vi "Zoe.prod.cons.vi"() -> ()   [LabVIEW 2014]
uses:
  Stack_State.ctl
  Stack Track.ctl
  Zoe_State.ctl
  PiFOC/PiFOC State.ctl
  <vilib>/vision/NI_Vision_Development_Module.lvlib
panel:
  in  "Move Piezo":bool
  out "Z Estimation":sgl(graph)
  in  "Template Path  2":path
  in  "Template Path":path
  out "Y Guess":dbl
  out "X Guess":dbl
  in  "Centroid Update":bool
  out "Cropped Image":T1(plugin-control)
  out "Raw Image":T1(plugin-control)
  in  "ROI Radius":dbl
  in  "Y Guess":dbl
  in  "X Guess":dbl
  out "Y Centroid":sgl
  out "X Centroid":sgl
  out "error out":errorcluster
  in  "stop":bool
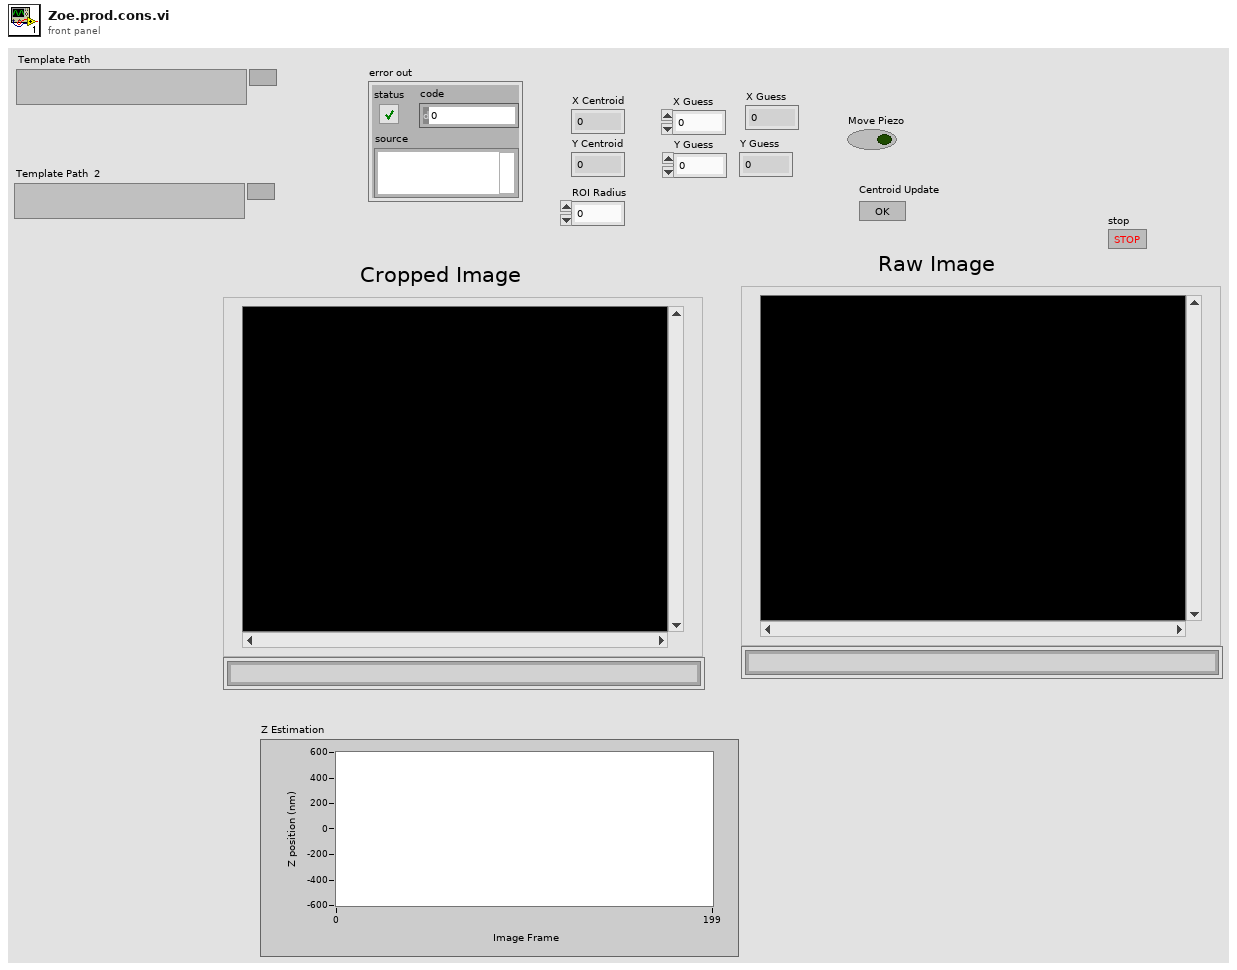
[diagram p1: front panel]
types:
  T1 = typedef "IMAQ Image.ctl" = refnum<image>
  T2 = typedef "PiFOC State.ctl" = enum16{"Idle", "GoTo", "getPosition"}
  T3 = typedef "Image Type" = u32
  T4 = typedef "Zoe_State.ctl" = enum16{"Centroid Update", "Idle", "Preview"}
  T5 = typedef "Stack_State.ctl" = cluster{"State":T6, "Stack Number":i32, "Image":u16[][], "Stacks":i32}
  T6 = typedef "Stack Track.ctl" = enum16{"Idle", "Preview", "Start Sequence", "Read Disk", "STOP", "Collecting", "End"}
  T7 = cluster{"Mean Value":sgl, "Standard Variation":sgl, "Minimal Value":sgl, "Maximal Value":sgl, "Area (calibrated)":sgl, "Area (pixels)":u32, "%":sgl, "Calibration Valid":bool}
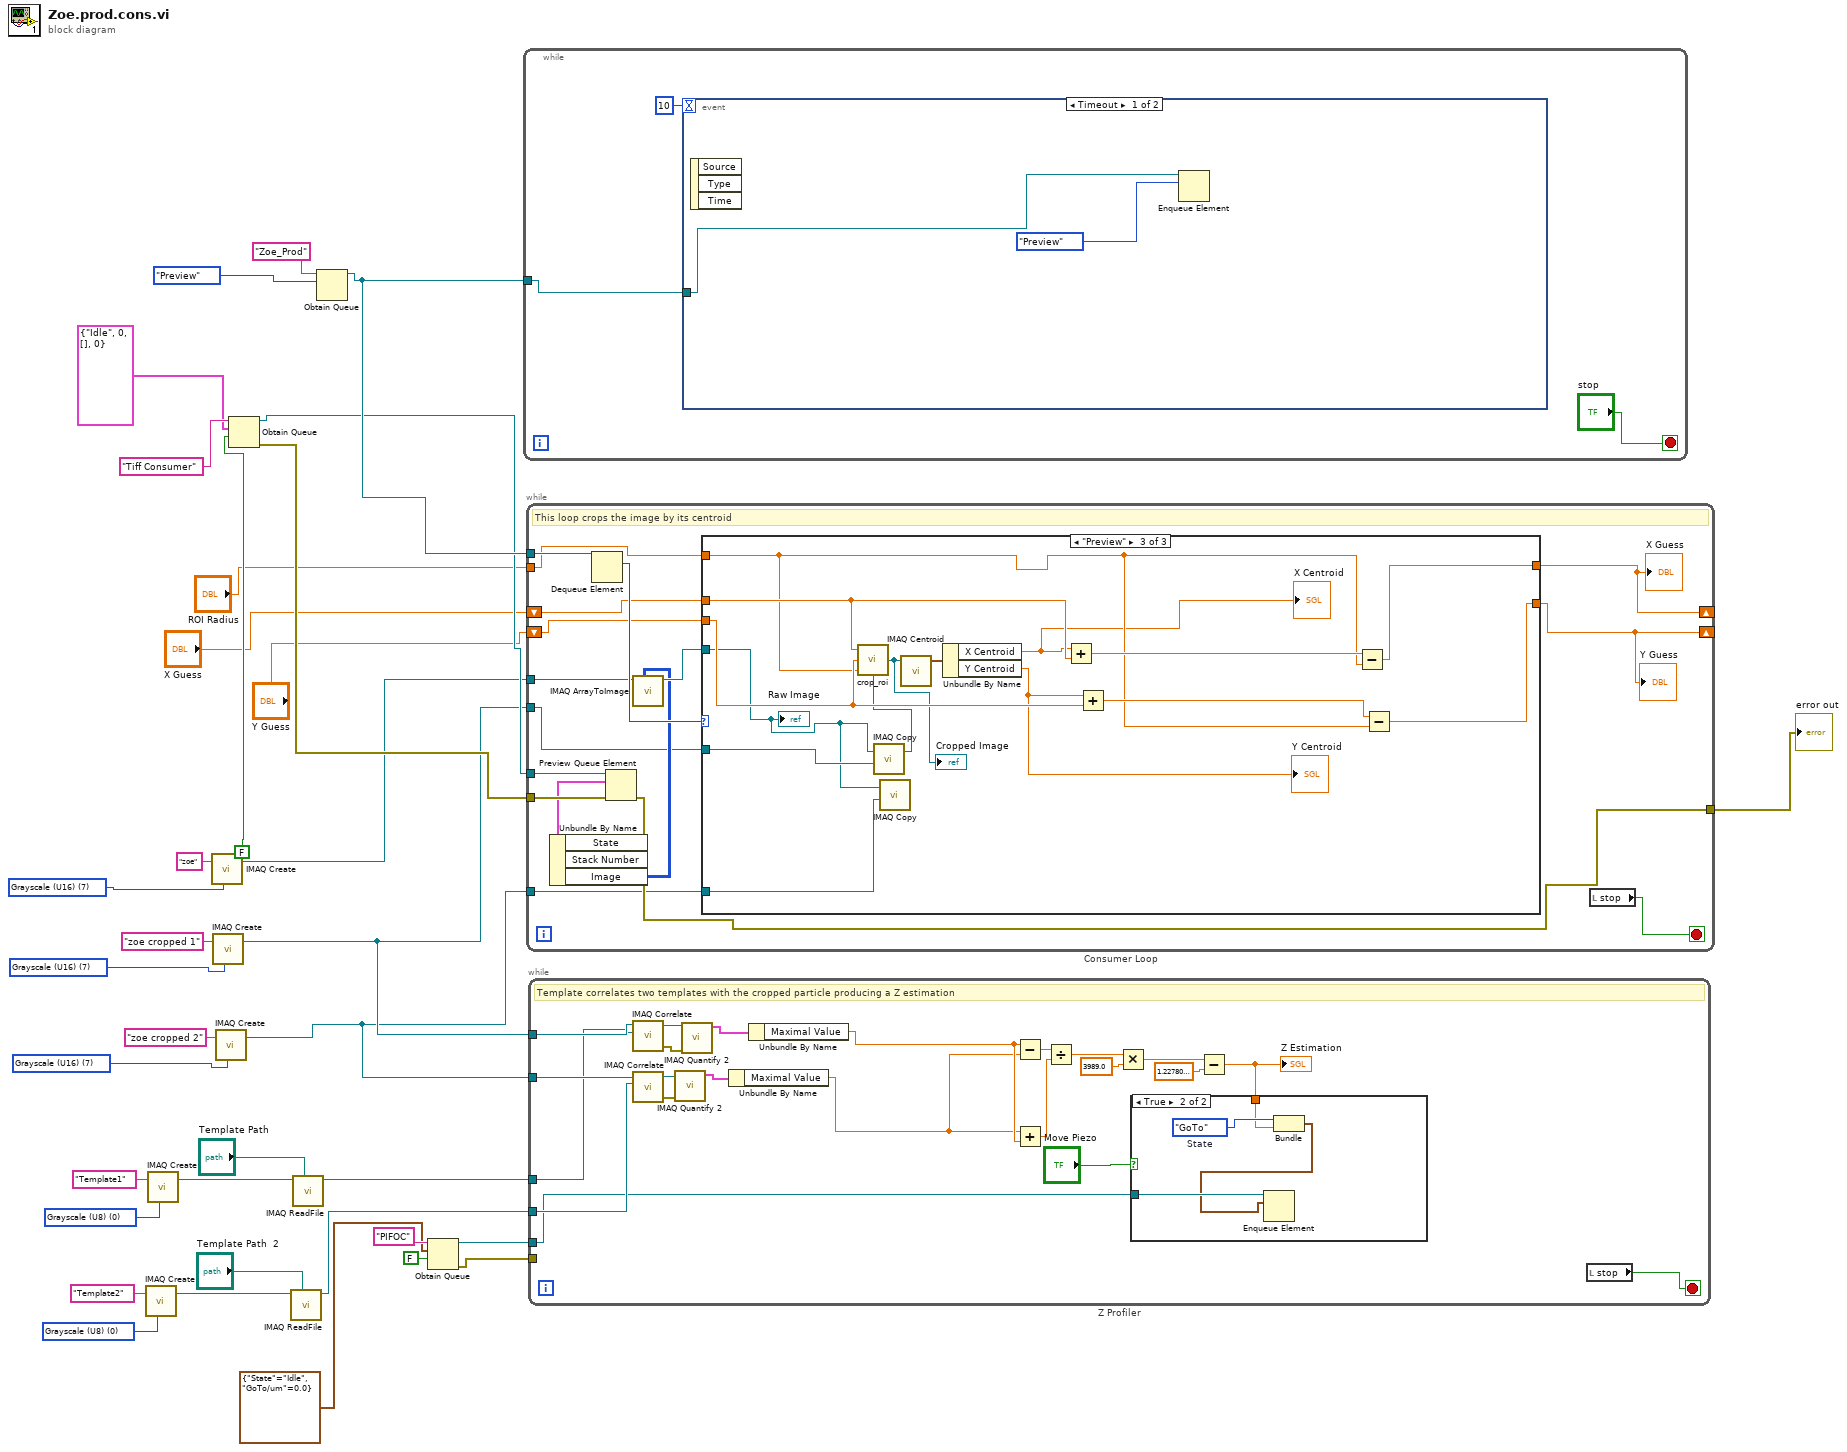
[diagram p0: block diagram]
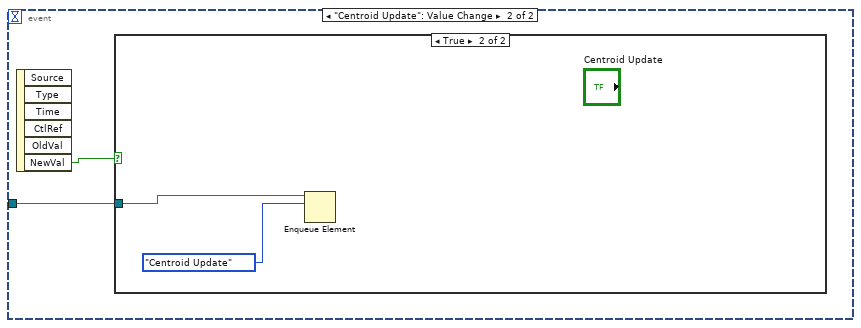
[diagram p5: hidden frame]
diagram:
  w8 = T3 0 items=["Grayscale (U8)", "Grayscale (I16)", "Grayscale (SGL)", "Complex (CSG)", "RGB (U32)", "HSL (U32)", "RGB (U64)", "Grayscale (U16)"] ("Image Type")
  w15 = T3 0 items=["Grayscale (U8)", "Grayscale (I16)", "Grayscale (SGL)", "Complex (CSG)", "RGB (U32)", "HSL (U32)", "RGB (U64)", "Grayscale (U16)"] ("Image Type")
  w18 = T3 7 items=["Grayscale (U8)", "Grayscale (I16)", "Grayscale (SGL)", "Complex (CSG)", "RGB (U32)", "HSL (U32)", "RGB (U64)", "Grayscale (U16)"] ("Image Type")
  w20 = T3 7 items=["Grayscale (U8)", "Grayscale (I16)", "Grayscale (SGL)", "Complex (CSG)", "RGB (U32)", "HSL (U32)", "RGB (U64)", "Grayscale (U16)"] ("Image Type")
  w23 = T3 7 items=["Grayscale (U8)", "Grayscale (I16)", "Grayscale (SGL)", "Complex (CSG)", "RGB (U32)", "HSL (U32)", "RGB (U64)", "Grayscale (U16)"] ("Image Type")
  n1 = call "IMAQ Create"("Image Name"="Template2", "Image Type"=w8) -> ("New Image"=w10:T1)  [unwired: 3 in, 1 out]
  n2 = call "IMAQ Create"("Image Name"="Template1", "Image Type"=w15) -> ("New Image"=w13:T1)  [unwired: 3 in, 1 out]
  n3 = call "IMAQ Create"("Image Name"="zoe", "Image Type"=w23) -> ("New Image"=w24:T1)  [unwired: 3 in, 1 out]
  n4 = call "IMAQ Create"("Image Name"="zoe cropped 1", "Image Type"=w20) -> ("New Image"=w19:T1)  [unwired: 3 in, 1 out]
  n5 = call "IMAQ Create"("Image Name"="zoe cropped 2", "Image Type"=w18) -> ("New Image"=w16:T1)  [unwired: 3 in, 1 out]
  n6 = Obtain Queue(name (unnamed)="Tiff Consumer", element data type=T5 {"State"=enum."Idle", "Stack Number"=0, "Image"=[], "Stacks"=0} ("input cluster"), create if not found? (T)=FALSE) -> (queue out=w30:refnum<queue>, error out=w29:errorcluster)  [unwired: 2 in, 1 out]
  n7 = call "IMAQ ReadFile"("File Path"="Template Path  2", "Image"=w10) -> ("Image Out"=w6:T1)  [unwired: 5 in, 4 out]
  n8 = call "IMAQ ReadFile"("File Path"="Template Path", "Image"=w13) -> ("Image Out"=w7:T1)  [unwired: 5 in, 4 out]
  n9 = Obtain Queue(name (unnamed)="Zoe_Prod", element data type=Zoe_State."Preview") -> (queue out=w31:refnum<queue>)  [unwired: 3 in, 2 out]
  n10 = Obtain Queue(name (unnamed)="PIFOC", element data type=cluster{"State":T2, "GoTo/um":dbl} {"State"=enum."Idle", "GoTo/um"=0.0} ("input cluster"), create if not found? (T)=FALSE) -> (queue out=w4:refnum<queue>, error out=w2:errorcluster)  [unwired: 2 in, 1 out]
  n11 = while {
    tunnel: w31 -> [w39]
    stop <- "stop" stop-if-true
    n12 = event shown="[0] Timeout" {
      selector: _ -> [_ _]
      dyn-events: _ -> [_ _]
      timeout: 10 -> [_ _]
      tunnel: w39 -> [w40 w42]
      event Timeout {
        n13 = event-data() -> ()  [unwired: 1 in, 3 out]
        n14 = Enqueue Element(queue=w40, element=Zoe_State."Preview") -> ()  [unwired: 2 in, 3 out]
      }
      event "Centroid Update": Value Change {
        n15 = event-data() -> ("NewVal"=w43:bool)  [unwired: 1 in, 5 out]
        n16 = case shown="True" w43 {
          tunnel: w42 -> [_ w45]
          frame False {
          }
          frame True {
            n17 = Enqueue Element(queue=w45, element=Zoe_State."Centroid Update") -> ()  [unwired: 2 in, 3 out]
          }
        }
      }
    }
  }
  n18 = while "Consumer Loop" {
    tunnel: w31 -> [w62]
    tunnel: w30 -> [w59]
    tunnel: w29 -> [w58]
    tunnel: "ROI Radius" -> [w55]
    shift-right: [w48] -> _
    shift-left: "Y Guess" -> [w56]
    shift-right: [w53] -> _
    shift-left: "X Guess" -> [w57]
    tunnel: w24 -> [w52]
    tunnel: [w51] -> w22
    tunnel: w19 -> [w47]
    tunnel: w16 -> [w46]
    stop <- w60 stop-if-true
    # "This loop crops the image by its centroid"
    n19 = Dequeue Element(queue=w62) -> (element=w61:T4)  [unwired: 2 in, 3 out]
    n20 = Preview Queue Element(queue=w59, error in (no error)=w58) -> (element=w50:T5, error out=w51:errorcluster)  [unwired: 1 in, 2 out]
    n21 = Unbundle By Name(w50) -> ("Image"=w49:u16[][])  [unwired: 2 out]
    n22 = call "IMAQ ArrayToImage"("Image Pixels (U16)"=w49, "Image"=w52) -> ("Image Out"=w54:T1)  [unwired: 8 in, 1 out]
    n23 = case shown="\"Preview\"" w61 {
      tunnel: w57 -> [w64 w66 w80]
      tunnel: w56 -> [w63 w65 w79]
      tunnel: w55 -> [_ _ w74]
      tunnel: w54 -> [_ _ w67]
      tunnel: [w64 w66 w77] -> w53
      tunnel: [w63 w65 w76] -> w48
      tunnel: w47 -> [_ _ w70]
      tunnel: w46 -> [_ _ w68]
      frame "Centroid Update", Default {
      }
      frame "Idle" {
      }
      frame "Preview" {
        n24 = call "IMAQ Copy"("Image Dst"=w70, "Image Src"=w67) -> ("Image Dst Out"=w71:T1)  [unwired: 4 in, 1 out]
        n25 = call "crop_roi.vi"("Refnum in"=w71, "Roy Radius"=w74, "Y"=w79, "X"=w80) -> ("Refnum in 2"=w69:T1)
        "Cropped Image" <- w69
        n26 = call "IMAQ Copy"("Image Dst"=w68, "Image Src"=w67) -> ()  [unwired: 4 in, 2 out]
        n27 = call "IMAQ Centroid"("Image"=w69) -> ("Centroid"=w81:cluster{"X Centroid":sgl, "Y Centroid":sgl})  [unwired: 3 in, 1 out]
        n28 = Unbundle By Name(w81) -> ("X Centroid"=w72:sgl, "Y Centroid"=w73:sgl)
        "X Centroid" <- w72
        "Y Centroid" <- w73
        n29 = Add(x=w72, y=w80) -> (x+y=w78:dbl)
        n30 = Add(x=w73, y=w79) -> (x+y=w75:dbl)
        n31 = Subtract(x=w78, y=w74) -> (x-y=w77:dbl)
        n32 = Subtract(x=w75, y=w74) -> (x-y=w76:dbl)
        "Raw Image" <- w67
      }
    }
    "X Guess" <- w53
    "Y Guess" <- w48
    n33 = local read "stop"() -> (w60:bool)
  }
  "error out" <- w22
  n34 = while "Z Profiler" {
    tunnel: w19 -> [w97]
    tunnel: w16 -> [w96]
    tunnel: w7 -> [w95]
    tunnel: w6 -> [w94]
    tunnel: w4 -> [w84]
    tunnel: w2 -> [_]
    stop <- w85 stop-if-true
    # "Template correlates two templates with the cropped particle producing a Z estimation"
    n35 = call "IMAQ Correlate"("Image Src"=w97, "Image Template"=w95) -> ("Image Dst Out"=w102:T1, "error out"=w103:errorcluster)  [unwired: 5 in]
    n36 = call "IMAQ Correlate"("Image Src"=w96, "Image Template"=w94) -> ("Image Dst Out"=w100:T1, "error out"=w101:errorcluster)  [unwired: 5 in]
    n37 = call "IMAQ Quantify 2"("error in (no error)"=w101, "Image"=w100) -> ("Global Report"=w98:T7)  [unwired: 7 in, 2 out]
    n38 = call "IMAQ Quantify 2"("error in (no error)"=w103, "Image"=w102) -> ("Global Report"=w99:T7)  [unwired: 7 in, 2 out]
    n39 = Unbundle By Name(w98) -> ("Maximal Value"=w86:sgl)
    n40 = Unbundle By Name(w99) -> ("Maximal Value"=w87:sgl)
    n41 = Subtract(x=w87, y=w86) -> (x-y=w88:sgl)
    n42 = Add(x=w86, y=w87) -> (x+y=w89:sgl)
    n43 = Divide(x=w88, y=w89) -> (x/y=w93:sgl)
    n44 = Multiply(x=w93, y=sgl 3989.0) -> (x*y=w91:sgl)
    n45 = Subtract(x=w91, y=sgl 1.2278) -> (x-y=w83:sgl)
    "Z Estimation" <- w83
    n46 = case shown="True" "Move Piezo" {
      tunnel: w84 -> [_ w107]
      tunnel: w83 -> [_ w105]
      frame False {
      }
      frame True {
        w106 = PiFOC_State."GoTo"  # State
        n47 = Bundle("State"=w106, w105) -> (w104:cluster{"State":T2, sgl})  [unwired: 1 in]
        n48 = Enqueue Element(queue=w107, element=w104) -> ()  [unwired: 2 in, 3 out]
      }
    }
    n49 = local read "stop"() -> (w85:bool)
  }
